vi "Get-client-channel-by-id.vi"(8 "error in (no error)":errorcluster, 10 "Client ID":i32, 11 "ModComm in":T1) -> (0 "error out":errorcluster, 2 "Client channels":refnum<queue>[](array[refnum]), 3 "ModComm out":T1)   [LabVIEW 2013, in "SLMServer.lvlib" / "SLMServer.lvclass"]
uses:
  SLMServer.lvclass
  Object-reference.ctl
  SA-SLMAPI/Sources/Message.lvclass
  SLMServer.lvclass/SLMServer.ctl
  Read Client channels.vi
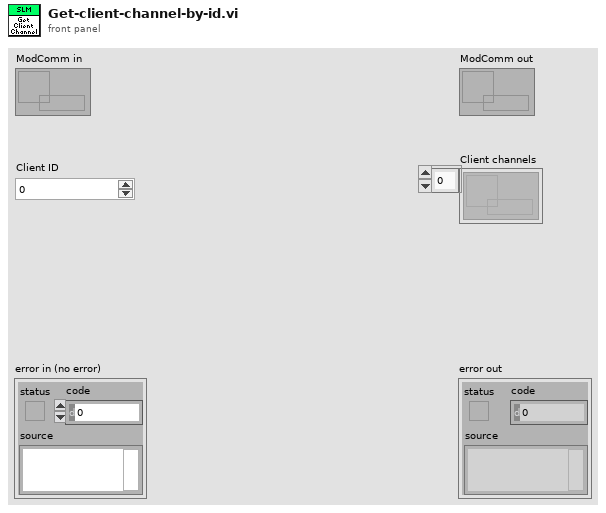
[diagram p1: front panel]
types:
  T1 = typedef "SLMServer.lvlib/SLMServer.lvclass/Object-reference.ctl" = refnum<data-value>
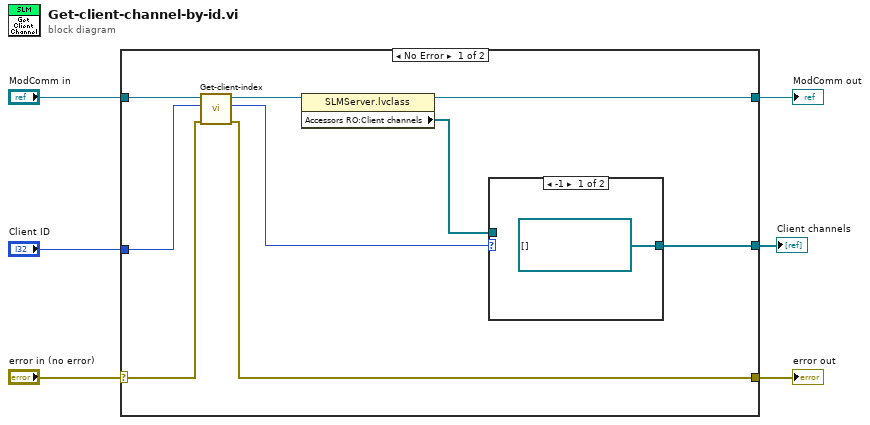
[diagram p0: block diagram]
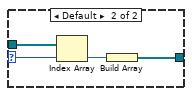
[diagram p2: hidden frame]
diagram:
  n1 = case shown="No Error" "error in (no error)" {
    selector: "error in (no error)" -> [w12 w22]
    tunnel: [w11 w22] -> w5
    tunnel: [w15 w21] -> w3
    tunnel: "ModComm in" -> [w14 w21]
    tunnel: "Client ID" -> [w10 _]
    tunnel: [w8 _] -> w1
    frame No Error {
      n2 = call "Get-client-index.vi"("error in (no error)"=w12, "Client ID"=w10, "ModComm in"=w14) -> ("error out"=w11:errorcluster, "Client index"=w7:i32, "ModComm out"=w13:T1)  [unwired: 6 in]
      n3 = property class="SLMServer.lvclass"(reference=w13) -> (reference out=w15:T1, "Accessors RO:Client channels"=w9:refnum<queue>[])  [unwired: 1 in, 1 out]
      n4 = case shown="-1" w7 {
        selector: w7 -> [_ w18]
        tunnel: w9 -> [_ w20]
        tunnel: [refnum<queue>[] [] ("Client channels") w17] -> w8
        frame -1 {
        }
        frame Default {
          n5 = Index Array(array=w20, index=w18) -> (element=w19:refnum<queue>)
          n6 = Build Array(w19) -> (w17:refnum<queue>[])
        }
      }
    }
    frame Error {
    }
  }
  "error out" <- w5
  "ModComm out" <- w3
  "Client channels" <- w1
